vi "trajectory_new_code_22_nov.vi"() -> ()   [LabVIEW 2019]
uses:
  <vilib>/FPGAPlugInAG/sbRIO-9629/niLvFpga_Open_sbRIO-9629.vi
  <vilib>/rvi/interface/common/dynamic/niFpgaDynamicAddResources.vi
  <vilib>/Utility/error.llb/Error Cluster From Error Code.vi
  <vilib>/rvi/errors/niLvFpgaAdjustHostInterfaceError.vi
  <vilib>/FPGAPlugInAG/Dynamic/niLvFpga_Close_Dynamic.vi
  <vilib>/rvi/interface/nirviOpenFPGA/nirviOpenFPGA.xnode
  FPGA Bitfiles/fcmsinglesection_FPGATarget_CloseLoopMotorTu_eGt+d+EV+VE.lvbitx
  Close_Loop_Motor_Tune.vi
  <vilib>/rvi/interface/nirviReadWriteControl/nirviReadWriteControl.xnode
  <vilib>/rvi/interface/nirviCloseFPGA/nirviCloseFPGA.xnode
  NiFpgaLv.dll
  <vilib>/rvi/interface/Simulation/niFpgaSimulationCallBeginRW.vi
panel:
  out "logical OR":bool
  out "Error":dbl[](array[numeric])
  in  "Kp":dbl[](array[numeric])
  out "Tip Position":dbl[](array[numeric])
  in  "radius":dbl=0.2
  in  "Degree Steps":dbl
  out "Current Tip Position":dbl[](array[numeric])
  out "data out":string
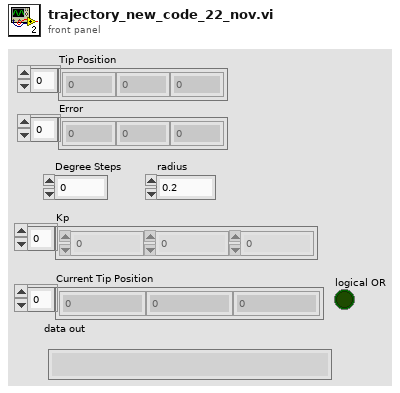
[diagram p1: front panel]
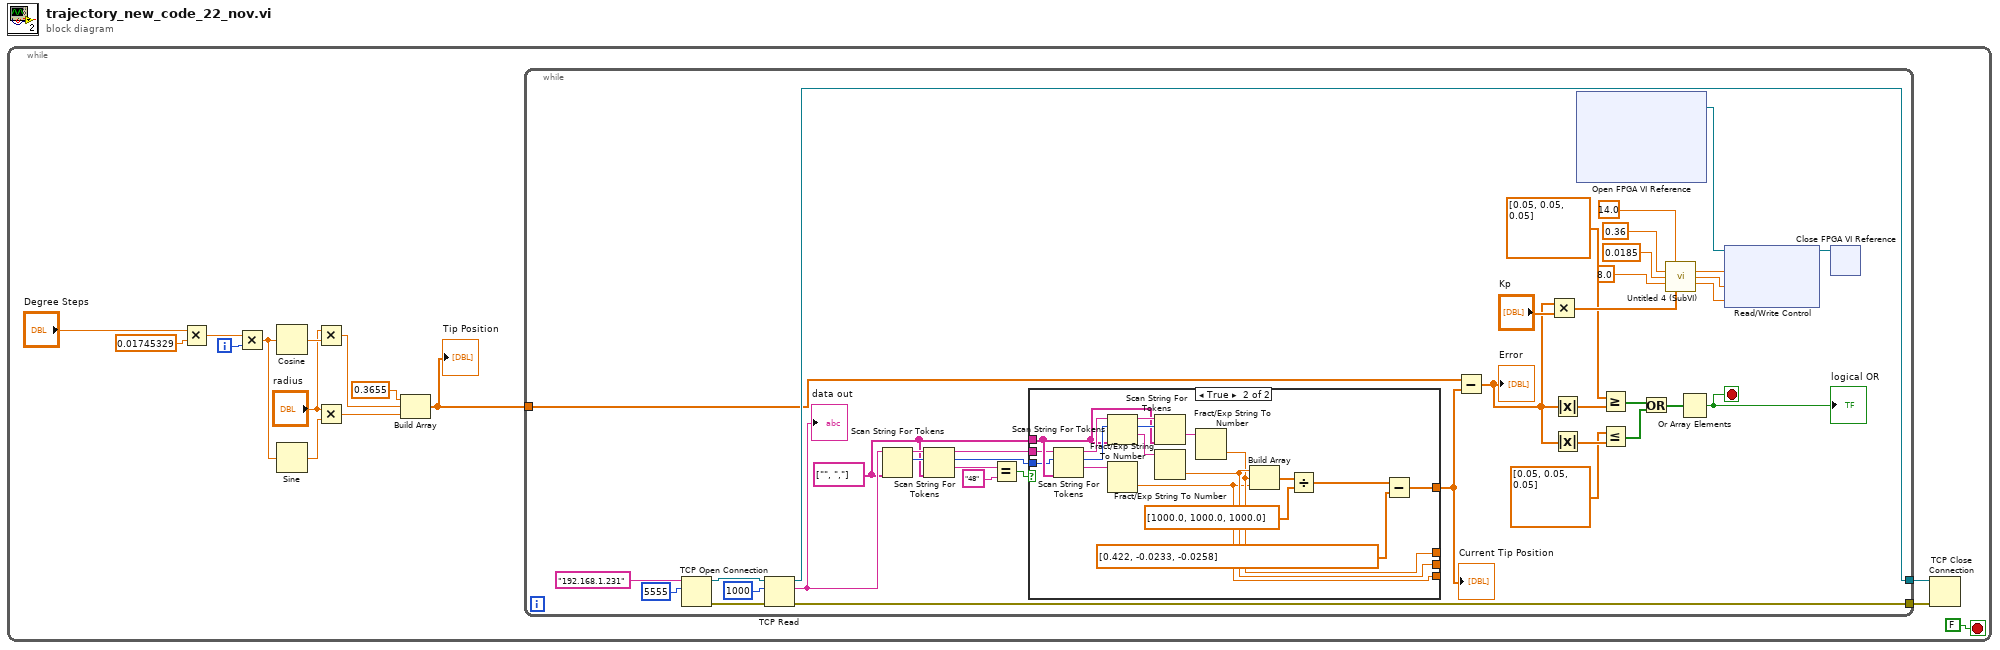
[diagram p0: block diagram]
diagram:
  n1 = while {
    i -> [w6]
    stop <- FALSE stop-if-true
    n2 = Multiply(x="Degree Steps", y=0.01745329) -> (x*y=w8:dbl)
    n3 = Multiply(x=w8, y=w6) -> (x*y=w11:dbl)
    n4 = Cosine(x=w11) -> (cos(x)=w13:dbl)
    n5 = Sine(x=w11) -> (sin(x)=w12:dbl)
    n6 = Multiply(x="radius", y=w13) -> (x*y=w4:dbl)
    n7 = Multiply(x="radius", y=w12) -> (x*y=w3:dbl)
    n8 = Build Array(0.3655 ("element"), w4, w3) -> (w2:dbl[])
    "Tip Position" <- w2
    n9 = while {
      tunnel: [w53] -> w15
      tunnel: [w52] -> w14
      tunnel: w2 -> [w27]
      stop <- w16 stop-if-true
      w44 = string[] ["", ","] ("delimiters (\\s,\\t,\\r,\\n)")
      n10 = TCP Open Connection(address="192.168.1.231", remote port or service name=u16 5555) -> (connection ID=w31:refnum<k5>, error out=w32:errorcluster)  [unwired: 3 in]
      n11 = TCP Read(connection ID=w31, bytes to read=1000, error in (no error)=w32) -> (connection ID out=w52:refnum<k5>, data out=w46:string, error out=w53:errorcluster)  [unwired: 2 in]
      "data out" <- w46
      n12 = Scan String For Tokens(6:w44, 9:w46) -> (2:w48:i32, 3:w49:string)  [unwired: 4 in, 2 out]
      n13 = Scan String For Tokens(6:w44, 8:w48, 9:w49) -> (1:w50:string, 2:w43:i32, 3:w42:string)  [unwired: 3 in, 1 out]
      n14 = Equal?(x=w50, y="48") -> (x = y?=w45:bool)
      n15 = case shown="True" w45 {
        tunnel: [_ w60] -> w28
        tunnel: [_ w59] -> _
        tunnel: [_ w58] -> _
        tunnel: [_ w57] -> _
        tunnel: w44 -> [_ w56]
        tunnel: w43 -> [_ w55]
        tunnel: w42 -> [_ w54]
        frame False {
        }
        frame True {
          n16 = Scan String For Tokens(6:w56, 8:w55, 9:w54) -> (1:w67:string, 2:w69:i32, 3:w71:string)  [unwired: 3 in, 1 out]
          n17 = Scan String For Tokens(6:w56, 8:w69, 9:w71) -> (1:w66:string, 2:w68:i32, 3:w70:string)  [unwired: 3 in, 1 out]
          n18 = Fract/Exp String To Number(string=w67) -> (number=w57:dbl)  [unwired: 3 in, 1 out]
          n19 = Scan String For Tokens(6:w56, 8:w68, 9:w70) -> (1:w65:string)  [unwired: 3 in, 3 out]
          n20 = Fract/Exp String To Number(string=w66) -> (number=w59:dbl)  [unwired: 3 in, 1 out]
          n21 = Fract/Exp String To Number(string=w65) -> (number=w58:dbl)  [unwired: 3 in, 1 out]
          n22 = Build Array(w59, w58, w57) -> (w64:dbl[])
          n23 = Divide(x=w64, y=dbl[] [1000.0, 1000.0, 1000.0]) -> (x/y=w62:dbl[])
          n24 = Subtract(x=w62, y=dbl[] [0.422, -0.0233, -0.0258]) -> (x-y=w60:dbl[])
        }
      }
      "Current Tip Position" <- w28
      n25 = Subtract(x=w27, y=w28) -> (x-y=w22:dbl[])
      "Error" <- w22
      n26 = Multiply(x=w22, y="Kp") -> (x*y=w25:dbl[])
      n27 = Absolute Value(x=w22) -> (abs(x)=w23:dbl[])
      n28 = Absolute Value(x=w22) -> (abs(x)=w21:dbl[])
      n29 = xnode "Open FPGA VI Reference"() -> ("FPGA VI Reference Out"=w41:refnum<k20>)  [unwired: 2 in, 1 out]
      n30 = Greater Or Equal?(x=dbl[] [0.05, 0.05, 0.05], y=w23) -> (x >= y?=w19:bool[])
      n31 = Less Or Equal?(x=dbl[] [0.05, 0.05, 0.05], y=w21) -> (x <= y?=w18:bool[])
      n32 = Or(x=w19, y=w18) -> (x .or. y?=w17:bool[])
      n33 = call "Untitled 4 (SubVI).vi"("Radius of motor pulley\n (mm)"=14.0 ("Radius of motor pulley\n (mm)"), "Length of the FCM (m)"=0.36, "Radius of disk (m)"=0.0185, "Number of Disks"=8.0, "Tip position Input"=w25) -> ("theta1"=w38:dbl, "theta2"=w37:dbl, "theta3"=w39:dbl)  [unwired: 2 in, 6 out]
      n34 = Or Array Elements(Boolean array=w17) -> (logical OR=w16:bool)
      "logical OR" <- w16
      n35 = xnode "Read/Write Control"("FPGA VI Reference In"=w41, "desired angle"=w38, "desired angle 2"=w37, "desired angle 3"=w39) -> ("FPGA VI Reference Out"=w40:refnum<k20>)  [unwired: 1 in, 1 out]
      n36 = xnode "Close FPGA VI Reference"("FPGA VI Reference In"=w40) -> ()  [unwired: 1 in, 1 out]
    }
    n37 = TCP Close Connection(connection ID=w14, error in (no error)=w15) -> ()  [unwired: 1 in, 2 out]
  }
